vi "串口接收.vi"() -> ()   [LabVIEW 2017]
uses:
  <vilib>/Instr/_visa.llb/VISA Flush IO Buffer Mask.ctl
  <vilib>/Instr/_visa.llb/VISA Configure Serial Port (Instr).vi
panel:
  out "read buffer":string
  in  "停止":bool
  out "波形图表":dbl(graph)
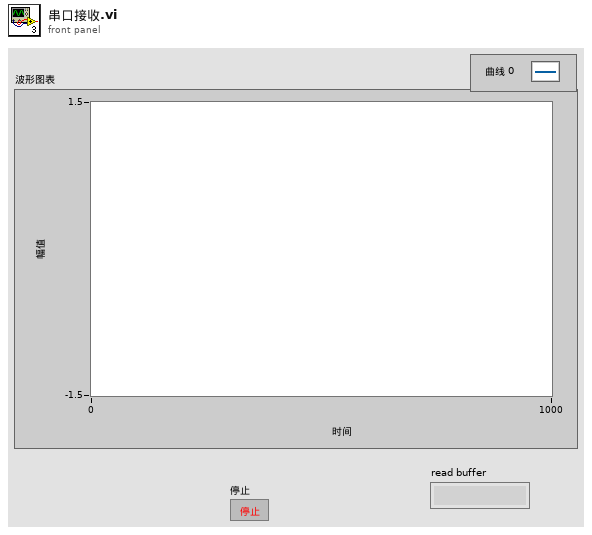
[diagram p1: front panel]
types:
  T1 = typedef "VISA Flush IO Buffer Mask.ctl" = u16
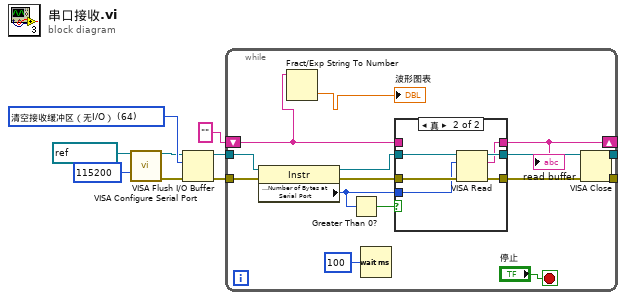
[diagram p0: block diagram]
diagram:
  w9 = T1 64 items=["清空接收缓冲区"=16, "向设备写入传输缓冲区"=32, "清空接收缓冲区（无I/O）"=64, "清空传输缓冲区"=128] ("Mask")
  n1 = call-poly "VISA Configure Serial Port"("VISA resource name"=refnum<visa-resource-name> "COM2", "baud rate (9600)"=u32 115200) -> ("VISA resource name out"=w7:refnum<visa-resource-name>, "error out"=w8:errorcluster)  [unwired: 12 in]
  n2 = VISA Flush I/O Buffer(VISA resource name=w7, mask (16)=w9, error in (no error)=w8) -> (VISA resource name out=w6:refnum<visa-resource-name>, error out=w5:errorcluster)
  n3 = while {
    tunnel: w6 -> [w23]
    tunnel: w5 -> [w22]
    tunnel: [w17] -> w4
    tunnel: [w16] -> w3
    shift-right: [w15] -> _
    shift-left: "" ("read buffer") -> [w12]
    stop <- "停止" stop-if-true
    n4 = property class="Instr"(reference=w23, error in=w22) -> (reference out=w20:refnum<visa-resource-name>, error out=w19:errorcluster, "Serial Settings:Number of Bytes at Serial Port"=w18:u32)
    n5 = Fract/Exp String To Number(string=w12) -> (number=→"波形图表":dbl)  [unwired: 3 in, 1 out]
    n6 = Greater Than 0?(x=w18) -> (x > 0?=w21:bool)
    n7 = Wait (ms)(milliseconds to wait=u32 100 ("等待时间（毫秒）")) -> ()  [unwired: 1 out]
    n8 = case shown="真" w21 {
      tunnel: w20 -> [w26 w32]
      tunnel: w19 -> [w25 w31]
      tunnel: w18 -> [_ w30]
      tunnel: [w26 w29] -> w17
      tunnel: [w25 w28] -> w16
      tunnel: [w24 w27] -> w15
      tunnel: w12 -> [w24 _]
      frame False {
      }
      frame True {
        n9 = VISA Read(VISA resource name=w32, byte count=w30, error in (no error)=w31) -> (VISA resource name out=w29:refnum<visa-resource-name>, read buffer=w27:string, error out=w28:errorcluster)  [unwired: 1 out]
      }
    }
    "read buffer" <- w15
  }
  n10 = VISA Close(VISA resource name=w4, error in (no error)=w3) -> ()  [unwired: 1 out]
